vi "Set gRPC ID.vi"(8 "error in":errorcluster, 10 "gRPC ID":T1, 11 "measurement plugin service in":refnum<class "Measurement Plugin Service.lvclass">) -> (0 "error out":errorcluster, 3 "measurement plugin service out":refnum<class "Measurement Plugin Service.lvclass">)   [LabVIEW 2021, in "NI Measurement Plug-In SDK.lvlib" / "Measurement Plugin Service.lvclass"]
uses:
  Measurement Plugin Service.lvclass
  <vilib>/gRPC/LabVIEW gRPC Library/Shared/grpcId.ctl
  Measurement Plugin Service.lvclass/Measurement Plugin Service.ctl
  <vilib>/gRPC/LabVIEW gRPC Library/grpc-lvsupport-release.lvlib
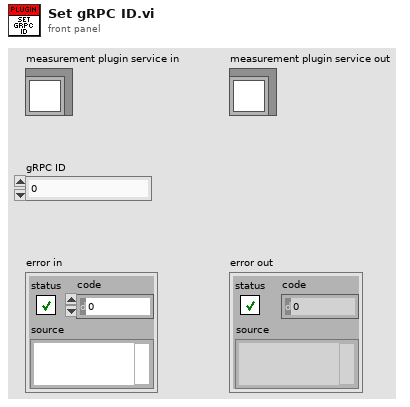
[diagram p1: front panel]
types:
  T1 = typedef "grpc-lvsupport-release.lvlib/grpcId.ctl" = u64
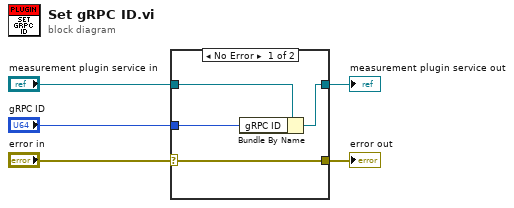
[diagram p0: block diagram]
diagram:
  n1 = case shown="No Error" "error in" {
    selector: "error in" -> [w9 w10]
    tunnel: [w9 w10] -> w4
    tunnel: [w7 w11] -> w2
    tunnel: "measurement plugin service in" -> [w8 w11]
    tunnel: "gRPC ID" -> [w6 _]
    frame No Error {
      n2 = Bundle By Name(cluster=w8, "gRPC ID"=w6) -> (w7:refnum<class "Measurement Plugin Service.lvclass">)
    }
    frame Error {
    }
  }
  "error out" <- w4
  "measurement plugin service out" <- w2
